vi "simple rw example.vi"() -> ()   [LabVIEW 2021]
uses:
  c4d05b1a-3696-4c59-8711-96d4ad6d8182.vi
  540b0a09-9276-4d5b-8447-d7098e6b937d.vi
  7170e333-48bf-49c2-83ae-a104c56fbe1d.vi
  57451aaa-aac1-47e8-8e78-d39de415d2c6.vi
  6bfd6412-5d24-477e-87a6-5ce7396f3706.vi
  0d6f7ce7-2490-4e2f-918f-7e287e999299.vi
  cebf75dc-e8e2-498d-a301-50682d0bdf83.vi
  f36fd5aa-1c2d-4d6b-8bd0-06edf8adb67b.vi
  46aa984f-ad87-48cc-a04c-773c6b1c6ff4.vi
  c4d05b1a-3696-4c59-8711-96d4ad6d8182.vi/49b3dd2d-4579-4089-b72e-3f0875c862f2.vi
  SubVIs/Check Error.vi
  SubVIs/Get Element Write Position.vi
  7170e333-48bf-49c2-83ae-a104c56fbe1d.vi/ad4ed45e-f2aa-403d-a38b-be52afbcecdf.vi
  57451aaa-aac1-47e8-8e78-d39de415d2c6.vi/49b3dd2d-4579-4089-b72e-3f0875c862f2.vi
  0d6f7ce7-2490-4e2f-918f-7e287e999299.vi/ad4ed45e-f2aa-403d-a38b-be52afbcecdf.vi
  cebf75dc-e8e2-498d-a301-50682d0bdf83.vi/bd07d5d9-1209-45ad-b636-9e9ab86132fb.vi
  46aa984f-ad87-48cc-a04c-773c6b1c6ff4.vi/ad4ed45e-f2aa-403d-a38b-be52afbcecdf.vi
  SubVIs/Set Element Read Position.vi
  SubVIs/Get Element Read Position.vi
  <vilib>/Utility/error.llb/Trim Whitespace.vi
  SubVIs/Get Element Description Variant.vi
  <vilib>/Utility/error.llb/Error Cluster From Error Code.vi
  SubVIs/Get Element Info Variant.vi
  SubVIs/Notify Of New Write.vi
  SubVIs/Wait For N Elements Available.vi
  CIF_NI_CIPC.lvlib
panel:
  out "Pass":bool
  out "element 2":dbl[](array[numeric])
  out "error out":errorcluster
  out "element":dbl
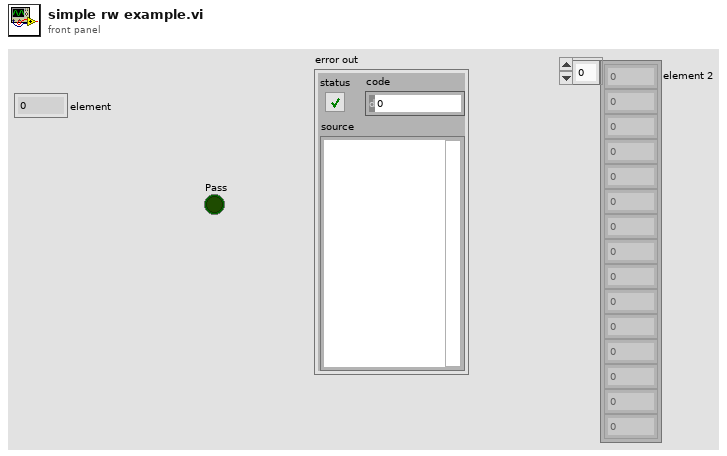
[diagram p1: front panel]
types:
  T1 = cluster{u16, "num":i32, bool, cluster{dbl, bool}}
  T2 = typedef "Read Result Details.ctl" = cluster{"Array Size":u32, "Element Offset Last Read":u32, "Overwritten":bool}
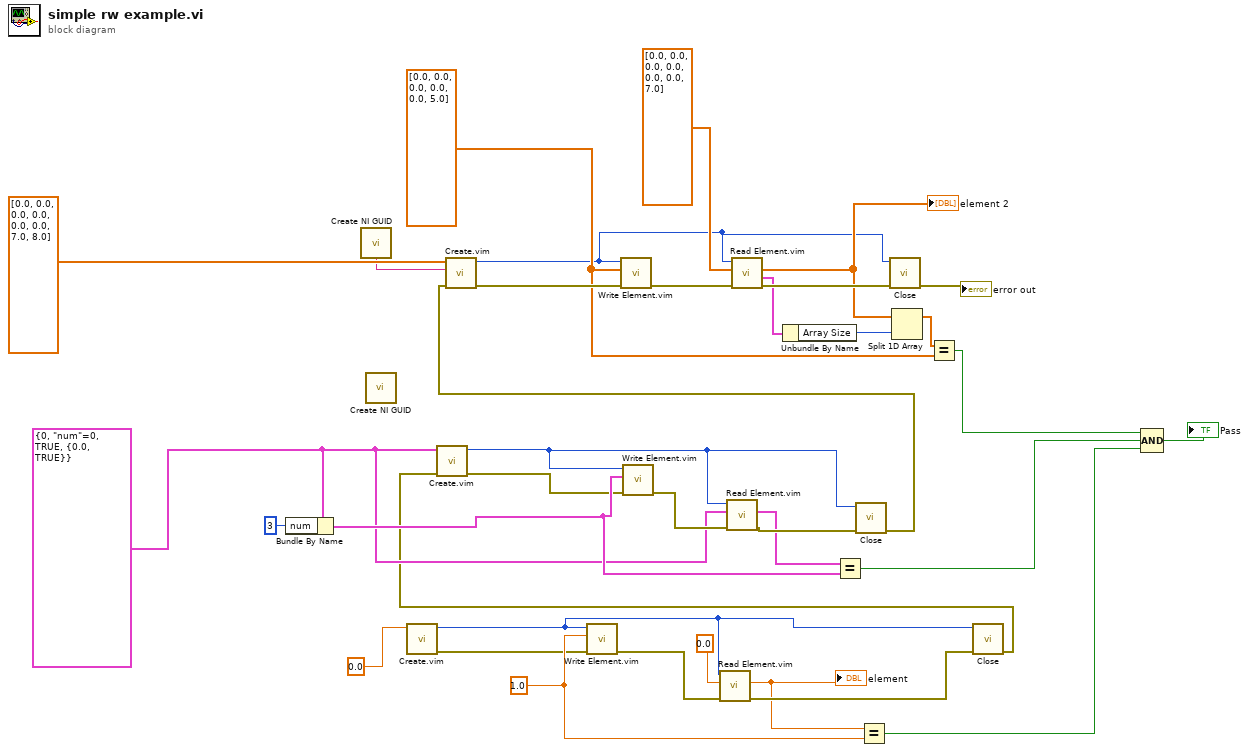
[diagram p0: block diagram]
diagram:
  w4 = dbl[] [0.0, 0.0, 0.0, 0.0, 0.0, 5.0]
  w11 = T1 {0, "num"=0, TRUE, {0.0, TRUE}}
  w7 = 1.0
  n1 = Bundle By Name(cluster=w11, "num"=3) -> (w33:T1)
  n2 = call <vilib>:"Create NI GUID.vi"() -> ("NI GUID"=w19:string)
  n3 = call <vilib>:"Create NI GUID.vi"() -> ()  [unwired: 1 out]
  n4 = call "Create.vim"("Data Type"=0.0) -> ("error out"=w6:errorcluster, "CIPC Reference"=w8:u64)  [unwired: 7 in, 2 out]
  n5 = call "Write Element.vim"("error in (no error)"=w6, "element"=w7, "CIPC Reference"=w8) -> ("error out"=w9:errorcluster)  [unwired: 6 in, 2 out]
  n6 = call "Read Element.vim"("error in"=w9, "Data in"=0.0, "CIPC Reference"=w8) -> ("error out"=w24:errorcluster, "Data out"=w17:dbl)  [unwired: 5 in, 2 out]
  "element" <- w17
  n7 = Equal?(x=w17, y=w7) -> (x = y?=w26:bool)
  n8 = call "Close.vi"("error in (no error)"=w24, "CIPC Reference"=w8) -> ("error out"=w10:errorcluster)  [unwired: 9 in]
  n9 = call "Create.vim"("error in (no error)"=w10, "Data Type"=w11) -> ("error out"=w13:errorcluster, "CIPC Reference"=w12:u64)  [unwired: 6 in, 2 out]
  n10 = call "Write Element.vim"("error in (no error)"=w13, "element"=w33, "CIPC Reference"=w12) -> ("error out"=w14:errorcluster)  [unwired: 6 in, 2 out]
  n11 = call "Read Element.vim"("error in"=w14, "Data in"=w11, "CIPC Reference"=w12) -> ("error out"=w35:errorcluster, "Data out"=w15:T1)  [unwired: 5 in, 2 out]
  n12 = Equal?(x=w15, y=w33) -> (x = y?=w27:bool)
  n13 = call "Close.vi"("error in (no error)"=w35, "CIPC Reference"=w12) -> ("error out"=w18:errorcluster)  [unwired: 9 in]
  n14 = call "Create.vim"("error in (no error)"=w18, "Name in"=w19, "Data Type"=dbl[] [0.0, 0.0, 0.0, 0.0, 0.0, 0.0, 7.0, 8.0]) -> ("error out"=w5:errorcluster, "CIPC Reference"=w2:u64)  [unwired: 5 in, 2 out]
  n15 = call "Write Element.vim"("error in (no error)"=w5, "element"=w4, "CIPC Reference"=w2) -> ("error out"=w1:errorcluster)  [unwired: 6 in, 2 out]
  n16 = call "Read Element.vim"("error in"=w1, "Data in"=dbl[] [0.0, 0.0, 0.0, 0.0, 0.0, 0.0, 7.0], "CIPC Reference"=w2) -> ("error out"=w32:errorcluster, "Read Result Details"=w23:T2, "Data out"=w21:dbl[])  [unwired: 5 in, 1 out]
  "element 2" <- w21
  n17 = Unbundle By Name(w23) -> ("Array Size"=w22:u32)
  n18 = call "Close.vi"("error in (no error)"=w32, "CIPC Reference"=w2) -> ("error out"=→"error out":errorcluster)  [unwired: 9 in]
  n19 = Split 1D Array(array=w21, index=w22) -> (first subarray=w29:dbl[])  [unwired: 1 out]
  n20 = Equal?(x=w29, y=w4) -> (x = y?=w28:bool)
  n21 = Compound Arithmetic op=AND(w28, w27, w26) -> (→"Pass":bool)
